vi "Gyro PID Back Color Stop.vi"(6 "Target angle":sgl, 7 "Threshold to Color":i32=1200, 8 "Threshold to slow":i32=1000, 9 "Min. speed":i32=40, 10 "Max. speed":i32=80, 11 "EV3 in":T1) -> (3 "EV3 out":T1)   [LabVIEW 2016]
uses:
  <vilib>/NXT/Subs/LVHSConnector.ctl
  <vilib>/NXT/LegoClasses/BrickReference/BrickReference.lvclass
  <vilib>/NXT/Block Support/NXT_OutputPort.ctl
  <vilib>/NXT/Block Support/NXT_InputPort.ctl
  <vilib>/NXT/NXTIO Xnodes/NXTIONodeSubVIs/LEGOResetMotors.vi
  <vilib>/NXT/Dual Mode Library/Motors/Rotation.vi
  <vilib>/NXT/Dual Mode Library/Sensors/EV3_Color_Reflect.vi
  <vilib>/NXT/NXTIO Xnodes/NXTIONodeSubVIs/NXTMotorSteeringOn.vi
  <vilib>/NXT/NXTIO Xnodes/NXTIONodeSubVIs/NXTStopMotors.vi
  <vilib>/NXT/Dual Mode Library/Waits/Wait_Num.vi
  <vilib>/NXT/NXTIO Xnodes/NXTIOXNode/NXTIO.xnode
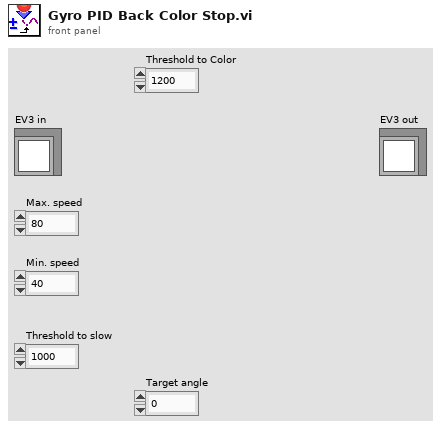
[diagram p1: front panel]
types:
  T1 = typedef "LVHSConnector.ctl" = refnum<class "BrickReference.lvclass">
  T2 = typedef "NXT_OutputPort.ctl" = u8
  T3 = typedef "NXT_InputPort.ctl" = u32
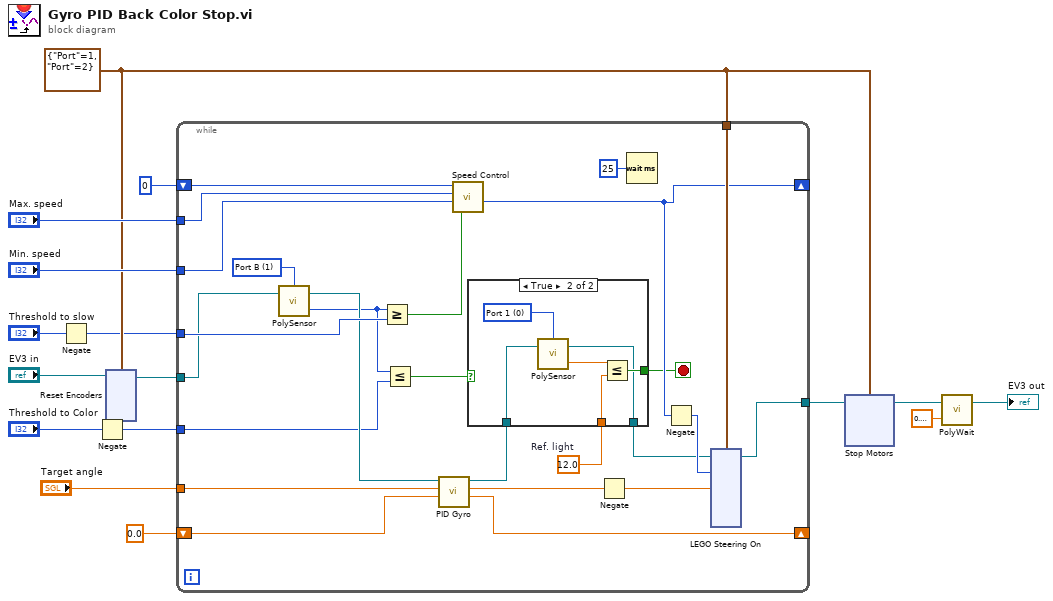
[diagram p0: block diagram]
diagram:
  w6 = cluster{"Port":T2, "Port":T2} {"Port"=1, "Port"=2} ("Motor")
  n1 = Negate(x="Threshold to slow") -> (-x=w2:i32)
  n2 = Negate(x="Threshold to Color") -> (-x=w1:i32)
  n3 = xnode "Reset Encoders"("Motors"=w6, "NXT/EV3"="EV3 in") -> ("NXT/EV3"=w12:T1)
  n4 = while {
    tunnel: w12 -> [w30]
    shift-right: [w41] -> _
    shift-left: sgl 0.0 -> [w26]
    tunnel: "Target angle" -> [w40]
    tunnel: [w37] -> w8
    tunnel: w6 -> [w39]
    shift-right: [w25] -> _
    shift-left: 0 -> [w34]
    tunnel: "Min. speed" -> [w31]
    tunnel: "Max. speed" -> [w33]
    tunnel: w2 -> [w32]
    tunnel: w1 -> [w24]
    stop <- w17 stop-if-true
    w18 = sgl 12.0  # Ref. light
    w38 = T2 1 items=["Port A", "Port B", "Port C", "Port D"] ("Port (Port A)")
    n5 = call-poly <vilib>:"PolySensor.vi"("NXT/EV3"=w30, "Port (Port A)"=w38) -> ("Angle of Rotation"=w27:i32, "NXT/EV3"=w29:T1)  [unwired: 1 in]
    n6 = Greater Or Equal?(x=w27, y=w32) -> (x >= y?=w28:bool)
    n7 = Less Or Equal?(x=w27, y=w24) -> (x <= y?=w21:bool)
    n8 = call "PID Gyro.vi"("Previous integral"=w26, "Target angle"=w40, "EV3 in"=w29) -> ("New integral"=w41:sgl, "Total error"=w35:sgl, "EV3 out"=w20:T1)  [unwired: 6 in]
    n9 = call "Speed Control.vi"("Speed Up or Down?"=w28, "Min. speed"=w31, "Max. speed"=w33, "Ini. speed"=w34) -> ("Speed out"=w25:i32)  [unwired: 7 in]
    n10 = case shown="True" w21 {
      tunnel: [_ w46] -> w17
      tunnel: w20 -> [w42 w45]
      tunnel: [w42 w44] -> w19
      tunnel: w18 -> [_ w43]
      frame False {
      }
      frame True {
        w48 = T3 0 items=["Port 1", "Port 2", "Port 3", "Port 4"] ("Port (Port 1)")
        n11 = call-poly <vilib>:"PolySensor.vi"("NXT/EV3"=w45, "Port (Port 1)"=w48) -> ("Scaled Value"=w47:sgl, "NXT/EV3"=w44:T1)  [unwired: 1 in]
        n12 = Less Or Equal?(x=w47, y=w43) -> (x <= y?=w46:bool)
      }
    }
    n13 = Negate(x=w35) -> (-x=w22:sgl)
    n14 = Wait (ms)(milliseconds to wait=u32 25) -> ()  [unwired: 1 out]
    n15 = Negate(x=w25) -> (-x=w23:i32)
    n16 = xnode "LEGO Steering On"("Steering 1"=w22, "Power 1"=w23, "Motors"=w39, "NXT/EV3"=w19) -> ("NXT/EV3"=w37:T1)
  }
  n17 = xnode "Stop Motors"("Motors"=w6, "NXT/EV3"=w8) -> ("NXT/EV3"=w7:T1)
  n18 = call-poly <vilib>:"PolyWait.vi"("Time (1 sec)"=sgl 0.2, "NXT/EV3"=w7) -> ("NXT/EV3"=→"EV3 out":T1)  [unwired: 2 in]
